vi "PrepareExtinctionCrossSectionToFile.vi"(0 "Extinction ExtinctionUncertainity Size parameter and Number ofS sizes":T4, 1 "RI results":T1, 2 "Particle Distribution Data":T3, 3 "Min Wavelength index":i32 min=0 max=150 step=1, 4 "Max Wavelength index":i32=20 min=0 max=150 step=1) -> (5 "Extinction":dbl[][](array[numeric]), 6 "CorrectedExtinction":dbl[][](array[numeric]), 7 "Sigma_diameter_string":string[](array[string]))   [LabVIEW 2013]
uses:
  ReadBaesDataTypeDefinition.ctl
  ParticleDistributionData.ctl
  BaesDataTypeDefinition.ctl
  RIandRIMCResults.ctl
panel:
  out "Sizes":dbl[](array[numeric])
  in  "Extinction ExtinctionUncertainity Size parameter and Number ofS sizes 2":T2={"Extinction"=[], "Extinction Uncertainty"=[], "Size parameters"=[], "Number ofSizes"=0.0, "GeometricCrossSection"=[], "Wave Length"=0.0, "SMPS Sizes"=[], "Concentration"=[], "Double Charge Correction"=FALSE, "Extincation Factor"=1.0, "Diameter Factor"=1.0, "Diameter Offset"=0.0, "Extinction Factor Flag"=FALSE, "Diameter Factor Flag"=FALSE, "Diameter Offset Flag"=FALSE, "Sizes"=[], "ExtinctionOrAbsorptionOrScattering"=0} {"ExtinctionOrAbsorptionOrScattering" scale=0.0..2.0}
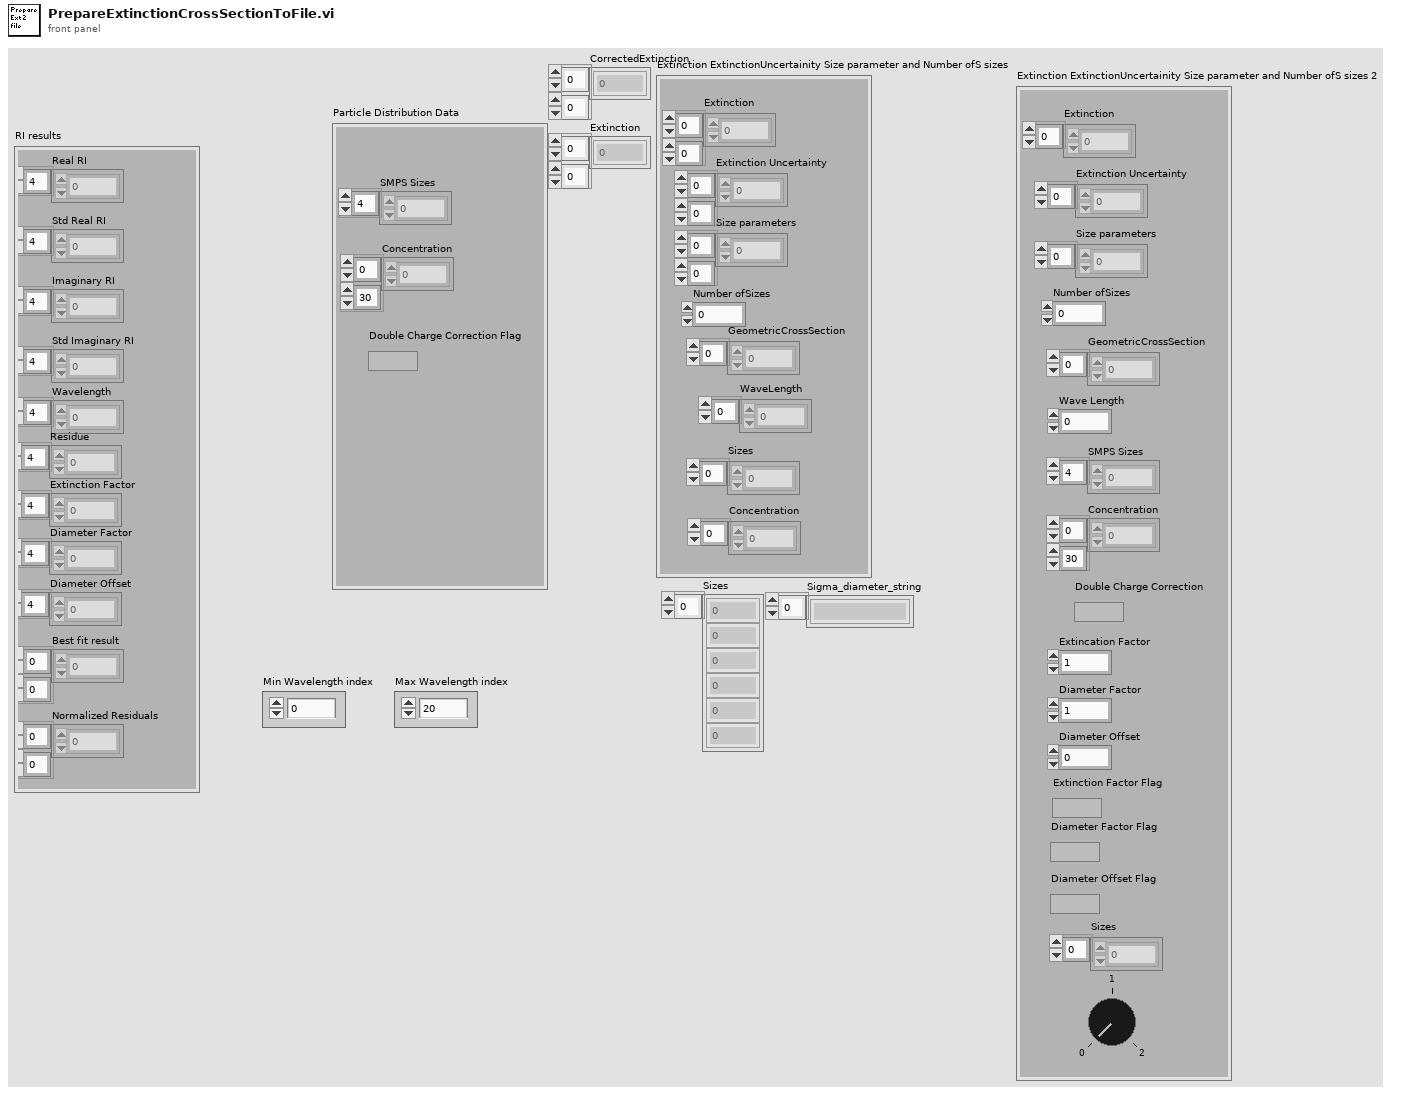
[diagram p1: front panel]
types:
  T1 = typedef "RIandRIMCResults.ctl" = cluster{"Real RI":dbl[], "Imaginary RI":dbl[], "Std Imaginary RI":dbl[], "Std Real RI":dbl[], "Wavelength":dbl[], "Residue":dbl[], "Extinction Factor":dbl[], "Diameter Factor":dbl[], "Diameter Offset":dbl[], "Best fit result":dbl[][], "Normalized Residuals":dbl[][]}
  T2 = typedef "BaesDataTypeDefinition.ctl" = cluster{"Extinction":dbl[], "Extinction Uncertainty":dbl[], "Size parameters":dbl[], "Number ofSizes":dbl, "GeometricCrossSection":dbl[], "Wave Length":dbl, "SMPS Sizes":dbl[], "Concentration":dbl[][], "Double Charge Correction":bool, "Extincation Factor":dbl, "Diameter Factor":dbl, "Diameter Offset":dbl, "Extinction Factor Flag":bool, "Diameter Factor Flag":bool, "Diameter Offset Flag":bool, "Sizes":dbl[], "ExtinctionOrAbsorptionOrScattering":i8}
  T3 = typedef "ParticleDistributionData.ctl" = cluster{"SMPS Sizes":dbl[], "Concentration":dbl[][], "Double Charge Correction Flag":bool}
  T4 = typedef "ReadBaesDataTypeDefinition.ctl" = cluster{"Extinction":dbl[][], "Extinction Uncertainty":dbl[][], "Size parameters":dbl[][], "Number ofSizes":dbl, "GeometricCrossSection":dbl[], "WaveLength":dbl[], "Sizes":dbl[], "Concentration":dbl[]}
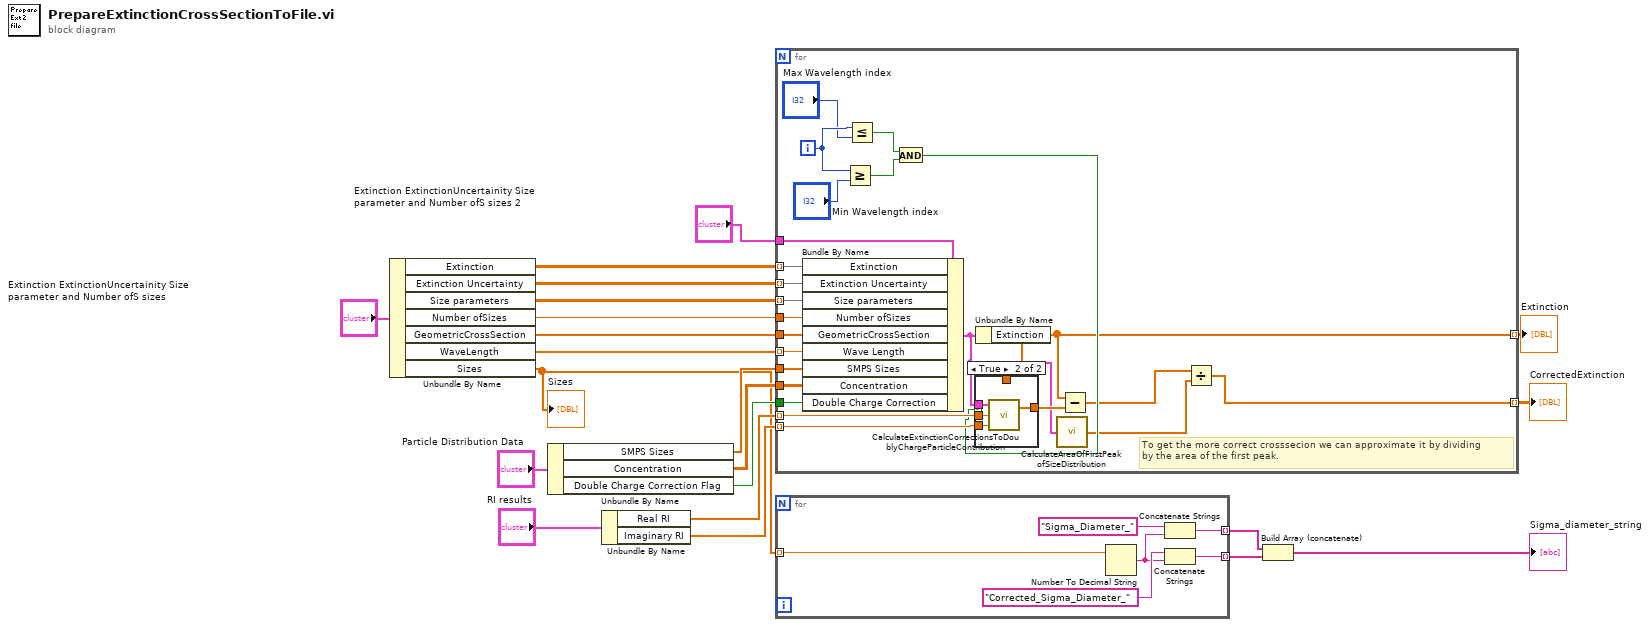
[diagram p0: block diagram]
diagram:
  n1 = Unbundle By Name("Extinction ExtinctionUncertainity Size parameter and Number ofS sizes") -> ("Extinction"=w13:dbl[][], "Extinction Uncertainty"=w12:dbl[][], "Size parameters"=w11:dbl[][], "Number ofSizes"=w20:dbl, "GeometricCrossSection"=w21:dbl[], "WaveLength"=w10:dbl[], "Sizes"=w4:dbl[])
  "Sizes" <- w4
  n2 = Unbundle By Name("Particle Distribution Data") -> ("SMPS Sizes"=w5:dbl[], "Concentration"=w17:dbl[][], "Double Charge Correction Flag"=w16:bool)
  n3 = Unbundle By Name("RI results") -> ("Real RI"=w7:dbl[], "Imaginary RI"=w6:dbl[])
  n4 = for {
    tunnel: [w26] -> w8 mode=indexing
    tunnel: w5 -> [w45]
    tunnel: w10 -> [w44] mode=indexing
    tunnel: w21 -> [w43]
    tunnel: w20 -> [w42]
    tunnel: w11 -> [w41] mode=indexing
    tunnel: w13 -> [w40] mode=indexing
    tunnel: w12 -> [w39] mode=indexing
    tunnel: w17 -> [w38]
    tunnel: w16 -> [w37]
    tunnel: "Extinction ExtinctionUncertainity Size parameter and Number ofS sizes 2" -> [w36]
    tunnel: [w22] -> w9 mode=indexing
    tunnel: w7 -> [w34] mode=indexing
    tunnel: w6 -> [w33] mode=indexing
    i -> [w30]
    # "To get the more correct crosssecion we can approximate it by dividing\nby the area of the first peak."
    n5 = Bundle By Name(cluster=w36, "Extinction"=w40, "Extinction Uncertainty"=w39, "Size parameters"=w41, "Number ofSizes"=w42, "GeometricCrossSection"=w43, "Wave Length"=w44, "SMPS Sizes"=w45, "Concentration"=w38, "Double Charge Correction"=w37) -> (w25:T2)
    n6 = Greater Or Equal?(x=w30, y="Min Wavelength index") -> (x >= y?=w31:bool)
    n7 = Less Or Equal?(x=w30, y="Max Wavelength index") -> (x <= y?=w28:bool)
    n8 = And(x=w28, y=w31) -> (x .and. y?=w27:bool)
    n9 = Unbundle By Name(w25) -> ("Extinction"=w26:dbl[])
    n10 = case shown="True" w27 {
      tunnel: w25 -> [_ w50]
      tunnel: [w46 w49] -> w35
      tunnel: w34 -> [_ w48]
      tunnel: w33 -> [_ w47]
      tunnel: w26 -> [w46 _]
      frame False {
      }
      frame True {
        n11 = call "CalculateExtinctionCorrectionsToDoublyChargeParticleContribution.vi"("refractive index, imaginary"=w47, "refractive index, real"=w48, "Extinction ExtinctionUncertainity Size parameter and Number ofS sizes"=w50) -> ("Expected Extinction Cross Section"=w49:sgl[])  [unwired: 1 out]
      }
    }
    n12 = call "CalculateAreaOfFirstPeakofSizeDistribution.vi"("Extinction ExtinctionUncertainity Size parameter and Number ofS sizes"=w25) -> ("Area of First peak"=w24:dbl[])
    n13 = Subtract(x=w26, y=w35) -> (x-y=w23:dbl[])
    n14 = Divide(x=w23, y=w24) -> (x/y=w22:dbl[])
  }
  "CorrectedExtinction" <- w9
  "Extinction" <- w8
  n15 = for {
    tunnel: w4 -> [w56] mode=indexing
    tunnel: [w54] -> w3 mode=indexing
    tunnel: [w51] -> w2 mode=indexing
    n16 = Number To Decimal String(number=w56) -> (decimal integer string=w52:string)  [unwired: 1 in]
    n17 = Concatenate Strings("Sigma_Diameter_", w52) -> (w54:string)
    n18 = Concatenate Strings("Corrected_Sigma_Diameter_", w52) -> (w51:string)
  }
  n19 = Build Array (concatenate)(w3, w2) -> (→"Sigma_diameter_string":string[])
